vi "WriteData.vi"(0 "Message":string, 1 "File Prefix":string, 2 "base path":path) -> ()   [LabVIEW 2011]
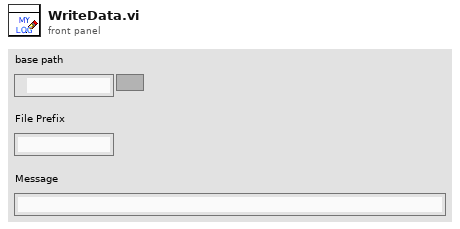
[diagram p1: front panel]
types:
  T1 = enum16{"open", "replace", "create", "open or create", "replace or create", "replace or create with confirmation"}
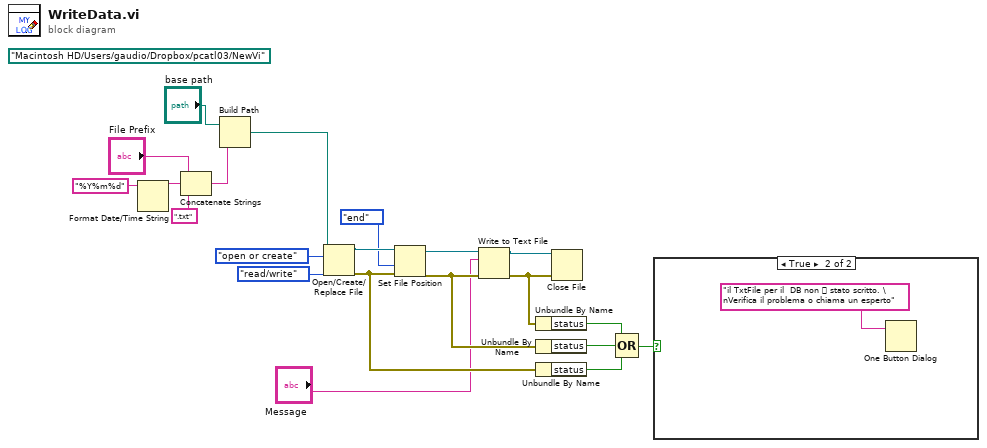
[diagram p0: block diagram]
diagram:
  (unwired) path "/Macintosh HD/Users/gaudio/Dropbox/pcatl03/NewVi" ("base path")
  n1 = Format Date/Time String(time format string (%c)="%Y%m%d") -> (date/time string=w14:string)  [unwired: 2 in]
  n2 = Concatenate Strings("File Prefix", w14, ".txt" ("string")) -> (w12:string)
  n3 = Build Path(base path="base path", name or relative path=w12) -> (appended path=w11:path)
  n4 = Open/Create/Replace File(file path (use dialog)=w11, operation (0:open)=T1."open or create", access (0:read/write)=enum16{"read/write", "read-only", "write-only"}."read/write") -> (refnum out=w18:refnum<file>, error out=w9:errorcluster)  [unwired: 3 in, 1 out]
  n5 = Set File Position(refnum=w18, from (0:start)=enum16{"start", "end", "current"}."end", error in=w9) -> (refnum out=w17:refnum<file>, error out=w8:errorcluster)  [unwired: 1 in]
  n6 = Write to Text File(file (use dialog)=w17, text="Message", error in=w8) -> (refnum out=w20:refnum<file>, error out=w10:errorcluster)  [unwired: 1 in, 1 out]
  n7 = Unbundle By Name(w10) -> ("status"=w7:bool)
  n8 = Unbundle By Name(w8) -> ("status"=w6:bool)
  n9 = Unbundle By Name(w9) -> ("status"=w5:bool)
  n10 = Close File(refnum=w20, error in=w10) -> ()  [unwired: 2 out]
  n11 = Compound Arithmetic op=OR(w7, w6, w5) -> (w4:bool)
  n12 = case shown="True" w4 {
    frame False {
    }
    frame True {
      n13 = One Button Dialog(message="il TxtFile per il  DB non  stato scritto. \nVerifica il problema o chiama un esperto") -> ()  [unwired: 1 in, 1 out]
    }
  }
